vi "Get Modem Status Digital Vars.vi"(0 "Common alarm handling(F)":bool, 11 "error in (no error)":errorcluster) -> (4 "Catagorised  Stsaus":T1[](array[typedef]), 6 "Values":T4[](array[typedef]), 8 "Analog Vars":T5[](array[typedef]), 10 "Any Alarm":bool, 13 "Primary Action":T3, 14 "Alarms":bool[](array[boolean]), 15 "error out":errorcluster)   [LabVIEW 2011]
uses:
  Digital GUI/Digital Display cluster.ctl
  Digital GUI/Digital Disp small indicator.ctl
  GUI/Status indicator white.ctl
  Status Digitalish.ctl
  Action List.ctl
  Catagorised alarm state.ctl
  GUI/Status Indikator Helper.ctl
  Action Analog Handler.ctl
  Tool/Variable List Tool Digital.ctl
  Common/Variable List Common Digital.ctl
  <vilib>/Utility/VariantDataType/GetNumericInfo.vi
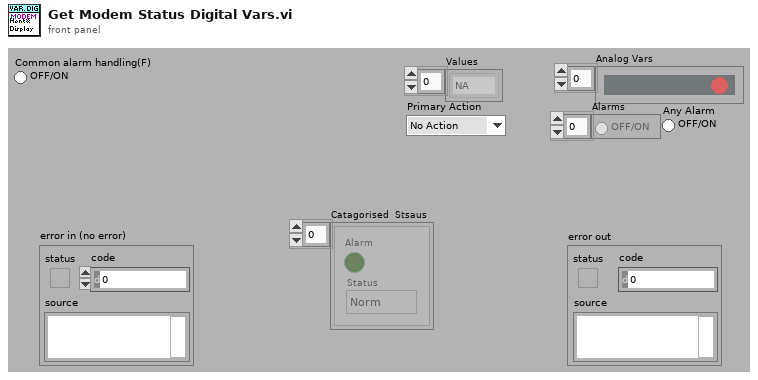
[diagram p1: front panel]
types:
  T1 = typedef "Catagorised alarm state.ctl" = cluster{"Alarm":bool, "Status":T2}
  T2 = typedef "Status Indikator Helper.ctl" = enum16{"Norm", "L", "H", "LL", "HH", "Value", "Technical"}
  T3 = typedef "Action List.ctl" = enum16{"No Action", "Stop Motor", "Turn Off HV"}
  T4 = typedef "Status Digitalish.ctl" = enum16{"NA", "False", "True"}
  T5 = typedef "Digital Display cluster.ctl" = cluster{"ON/OFF TEXT":string, "Val":T6, "Status":T7}
  T6 = typedef "Digital Disp small indicator.ctl" = u16
  T7 = typedef "Status indicator white.ctl" = u16
  T8 = typedef "Action Analog Handler.ctl" = enum16{"GET value", "GET Single Frequenzy", "GET All Values", "GET Waveform", "Get Numb Var", "SET Value", "START Buffer", "REG Variable", "BUF size(total antal sekund)", "PULS", "Get a Value at time", "Set initial waveform"}
  T9 = typedef "Variable List Tool Digital.ctl" = enum16{"Tool Error Controller", "Tool Stopped Controller", "Tool Relay 1", "Tool Relay 2", "Tool Both Relays", "Tool node Pressure 1", "Tool Error Pressure 1", "Tool Stopped Pressure 1", "Tool node Pressure 2", "Tool Error Pressure 2", "Tool Stopped Pressure 2", "Tool node Solenoid", "Tool Error Solenoid", "Tool Stopped Solenoid", "Tool Solenoid 1", "Tool Solenoid 2", "Tool Solenoid 3", "Tool node PSU", "Tool Error PSU", "Tool Stopped PSU", "Upper Tension Sub", "Tool Error Upper Tension Sub", "Tool Stopped Upper Tension Sub", "Lower Tension Sub", "Tool Error Lower Tension Sub", "Tool Stopped Lower Tension Sub", "Stroke Target seeking", "Stroke Moving Out", "Stroke Moving Inn", "Stroke valves set for Out", "Stroke valves set for In", "Stroke In (force)", "Stroke Out (force)", "Stroke Force decreasing(in)", "Stroke Force decreasing(out)", "Stroke Force change not correct", "Stroke SLIPS established P1", "Stroke SLIPS established P2", "Stroke SLIPS established", "Stroke Pressure Monitor Ongoing", "Stroke Pressure Monitor Ending ", "Tool Stroke enable Valve", "Tool Stroke direction Valve", "Tool Anchor Valve", "Stroker Var19 - Reserved", "Stroker Var20 - Reserved", "Stroker Var21 - Reserved", "Stroker Var22 - Reserved", "Stroker Var23 - Reserved", "Stroker Var24 - Reserved", "Tractor Var1 - Reserved", "Tractor Var2 - Reserved", "Tractor Var3 - Reserved", "Tractor Var4 - Reserved", "Tractor Var5 - Reserved", "Tractor Var6 - Reserved", "Tractor Var7 - Reserved", "Tractor Var8 - Reserved", "Oil filling mode", "Mill Bit Direction", "Position control", "Anchor", "Driller Var5 - Reserved", "Driller Var6 - Reserved", "Driller Var7 - Reserved", "Driller Var8 - Reserved"}
  T10 = typedef "Variable List Common Digital.ctl" = enum16{"PCP Connected", "PCP PC Control", "HV PSU connected", "HV PSU HV Active", "Modem Connected", "Tool Connected", "CanBus interface"}
  T11 = typedef "User Setting DigitalChannel.ctl" = cluster{"Responses":cluster{"Technical Error (NA)":T12, "OFF / FALSE":T13, "ON / TRUE":T13}}
  T12 = typedef "Alarm Responce.ctl" = cluster{"Action":T3, "Alarm":bool}
  T13 = typedef "Alarm Responce dig.ctl" = cluster{"Action":T3, "Alarm":bool, "Exclamation":bool}
  T14 = typedef "Fixed Digital Channel Definition.ctl" = cluster{"ID":u16, "Name":string, "NA Text":string, "Off Text":string, "On Text":string, "Maximum upd":T15, "Comment":string, "Help file Name":string, "Help file Section ":string, "Catagory":T16, "In use":bool}
  T15 = typedef "Update frequensies.ctl" = enum16{"2 Hz", "1 Hz", "0.1 Hz"}
  T16 = typedef "Channel catagory Enum.ctl" = enum16{"No Category", "Power", "Temperature", "Pressure"}
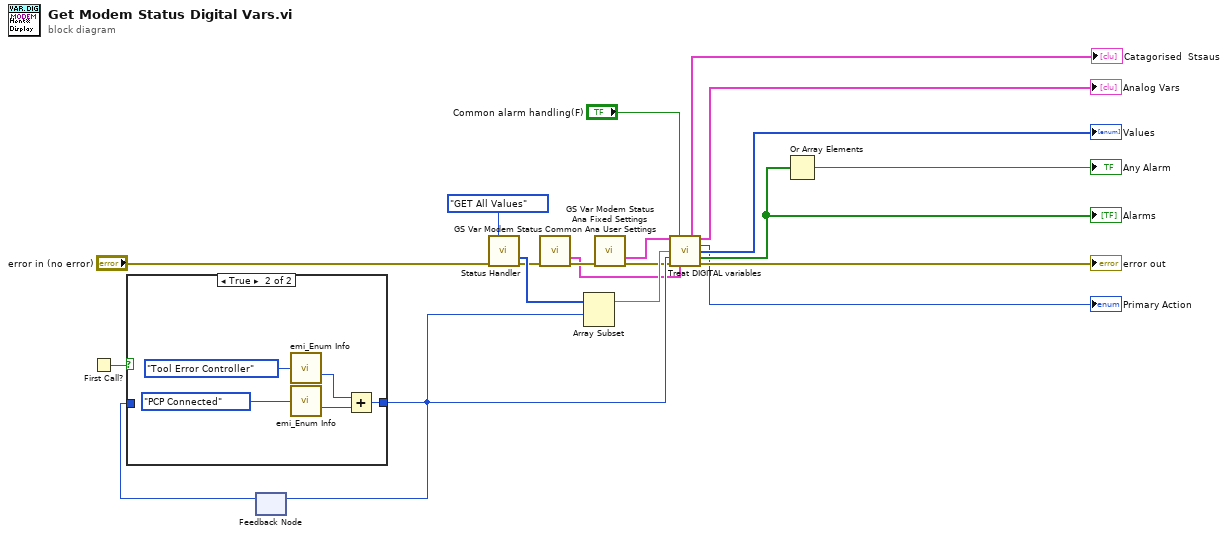
[diagram p0: block diagram]
diagram:
  n1 = First Call?() -> (First Call?: T/F=w8:bool)
  n2 = feedback #1() -> (w7:i32)  [unwired: 1 in]
  n3 = case shown="True" w8 {
    tunnel: [w21 w23] -> w6
    tunnel: w7 -> [w21 _]
    frame False {
    }
    frame True {
      n4 = call "emi_Enum Info.vi"("Enum"=Variable_List_Tool_Digital."Tool Error Controller" ("Variable")) -> ("Numb Elements"=w22:i32)  [unwired: 11 in, 3 out]
      n5 = call "emi_Enum Info.vi"("Enum"=Variable_List_Common_Digital."PCP Connected" ("Action")) -> ("Numb Elements"=w24:i32)  [unwired: 11 in, 3 out]
      n6 = Add(x=w22, y=w24) -> (x+y=w23:i32)
    }
  }
  n7 = feedback-in #1(w6) -> ()
  n8 = call "Status Handler.vi"("Action"=Action_Analog_Handler."GET All Values" ("Action(GET)"), "error in (no error)"="error in (no error)") -> ("Values"=w10:T4[], "error out"=w2:errorcluster)  [unwired: 9 in, 3 out]
  n9 = call "GS Var Modem Status Common Ana User Settings.vi"("error in (no error)"=w2) -> ("Modem Status digital var User settigns out"=w4:T11[], "error out"=w5:errorcluster)  [unwired: 12 in, 1 out]
  n10 = Array Subset(array=w10, index=w6) -> (w11:T4[])  [unwired: 1 in]
  n11 = call "GS Var Modem Status Ana Fixed Settings.vi"("error in (no error)"=w5) -> ("Modem Status Digital Var Fixed out"=w3:T14[], "error out"=w1:errorcluster)  [unwired: 12 in, 1 out]
  n12 = call "Treat DIGITAL variables.vi"("Analog Variable info fixed"=w3, "Common alarm handling(F)"="Common alarm handling(F)", "Status Values"=w11, "Variabel start index"=w6, "error In"=w1, "Analog Variable info Settings"=w4) -> ("Categorized  Status"=→"Catagorised  Stsaus":T1[], "Digital Variable Display"=→"Analog Vars":T5[], "Action"=→"Primary Action":T3, "Digital status Values"=→"Values":T4[], "Alarms"=w19:bool[], "error out"=→"error out":errorcluster)  [unwired: 3 in, 1 out]
  "Alarms" <- w19
  n13 = Or Array Elements(Boolean array=w19) -> (logical OR=→"Any Alarm":bool)
